vi "Phase control start (SubVI).vi"(0 "VISA Refnum in":refnum<visa-resource-name>, 1 "pos_z_in":dbl, 2 "pos_xy_in":cluster{"pos_y":dbl, "pos_x":dbl}, 11 "error in":errorcluster) -> (4 "pos_no_sample":dbl, 6 "pos_sample":dbl, 8 "pos_z_out":dbl, 10 "pos_xy_out":cluster{"pos_y":dbl, "pos_x":dbl}, 13 "Profile_ns out":cluster{dbl[], dbl[]}, 14 "Profile_s out":cluster{dbl[], dbl[]}, 15 "error out":errorcluster)   [LabVIEW 2018]
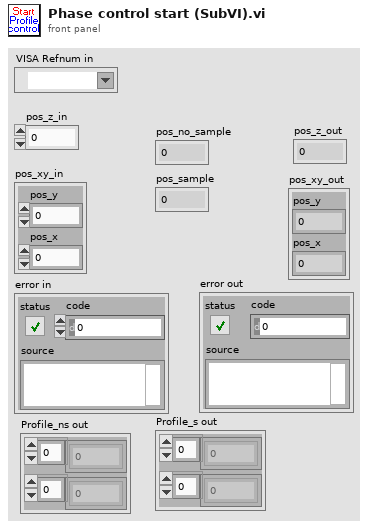
[diagram p1: front panel]
types:
  T1 = cluster{"pos_n":dbl, "pos_s":dbl, "pos_z":dbl, "pos_xy 2":cluster{"pos_x":dbl, "pos_y":dbl}, "Profile_ns out":cluster{dbl[], dbl[]}, "Profile_s out":cluster{dbl[], dbl[]}, "error out result":errorcluster}
  T2 = enum32{"Invalid", "Standard", "Closed", "Hidden", "Minimized", "Maximized"}
  T3 = cluster{"pos_z_in":dbl, "VISA Refnum in":refnum<visa-resource-name>, "pos_xy_in":cluster{"pos_y":dbl, "pos_x":dbl}}
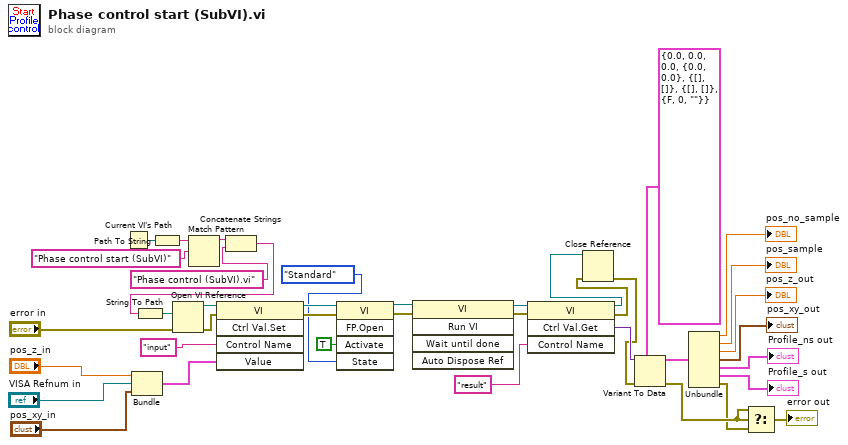
[diagram p0: block diagram]
diagram:
  n1 = Current VI's Path() -> (path=w17:path)
  n2 = Bundle("pos_z_in"="pos_z_in", "VISA Refnum in"="VISA Refnum in", "pos_xy_in"="pos_xy_in") -> (w28:T3)  [unwired: 1 in]
  n3 = Path To String(path=w17) -> (string=w24:string)
  n4 = Match Pattern(string=w24, regular expression="Phase control start (SubVI)") -> (before substring=w19:string)  [unwired: 1 in, 3 out]
  n5 = Concatenate Strings(w19, "Phase control (SubVI).vi") -> (w25:string)
  n6 = String To Path(string=w25) -> (path=w21:path)
  n7 = Open VI Reference(vi path=w21, error in (no error)="error in") -> (vi reference=w29:refnum<vi>, error out=w30:errorcluster)  [unwired: 1 in, 3 out]
  n8 = invoke class="VI" method="Ctrl Val.Set"(reference=w29, error in=w30, "Control Name"="input", "Value"=w28) -> (reference out=w34:refnum<vi>, error out=w33:errorcluster)  [unwired: 1 in, 3 out]
  n9 = invoke class="VI" method="FP.Open"(reference=w34, error in=w33, "Activate"=TRUE, "State"=T2."Standard") -> (reference out=w36:refnum<vi>, error out=w35:errorcluster)  [unwired: 1 in, 3 out]
  n10 = invoke class="VI" method="Run VI"(reference=w36, error in=w35) -> (reference out=w38:refnum<vi>, error out=w37:errorcluster)  [unwired: 3 in, 3 out]
  n11 = invoke class="VI" method="Ctrl Val.Get"(reference=w38, error in=w37, "Control Name"="result") -> (reference out=w9:refnum<vi>, error out=w8:errorcluster, "Get Control Value Variant"=w39:variant)  [unwired: 1 in, 1 out]
  n12 = Close Reference(reference=w9, error in (no error)=w8) -> (error out=w7:errorcluster)
  n13 = Variant To Data(error in=w7, type=T1 {"pos_n"=0.0, "pos_s"=0.0, "pos_z"=0.0, "pos_xy 2"={"pos_x"=0.0, "pos_y"=0.0}, "Profile_ns out"={[], []}, "Profile_s out"={[], []}, "error out result"={"status"=FALSE, "code"=0, "source"=""}} ("result"), Variant=w39) -> (data=w16:T1, error out=w15:errorcluster)
  n14 = Unbundle(w16) -> ("pos_n"=→"pos_no_sample":dbl, "pos_s"=→"pos_sample":dbl, "pos_z"=→"pos_z_out":dbl, "pos_xy 2"=→"pos_xy_out":cluster{"pos_x":dbl, "pos_y":dbl}, "Profile_ns out"=→"Profile_ns out":cluster{dbl[], dbl[]}, "Profile_s out"=→"Profile_s out":cluster{dbl[], dbl[]}, "error out result"=w5:errorcluster)
  n15 = Select(t=w15, s=w15, f=w5) -> (s? t:f=→"error out":errorcluster)
